vi "Save_Log_File(Subvi).vi"(0 "TX_Station":i32, 1 "RX_Station":i32, 3 "1D data":i32[](array[numeric]) caption="1D 데이터") -> (8 "참조 번호 출력":refnum<file>)   [LabVIEW 2024]
uses:
  <vilib>/Utility/sysdir.llb/System Directory Type.ctl
  <vilib>/Utility/file.llb/Write Delimited Spreadsheet (I64).vi
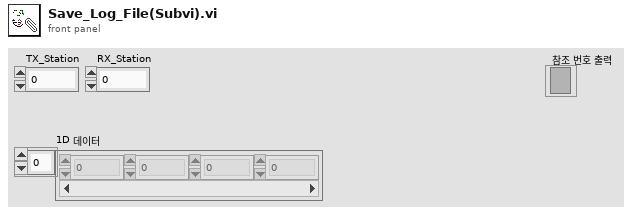
[diagram p1: front panel]
types:
  T1 = enum16{"open", "replace", "create", "open or create", "replace or create", "replace or create with confirmation"}
  T2 = typedef "System Directory Type.ctl" = i32
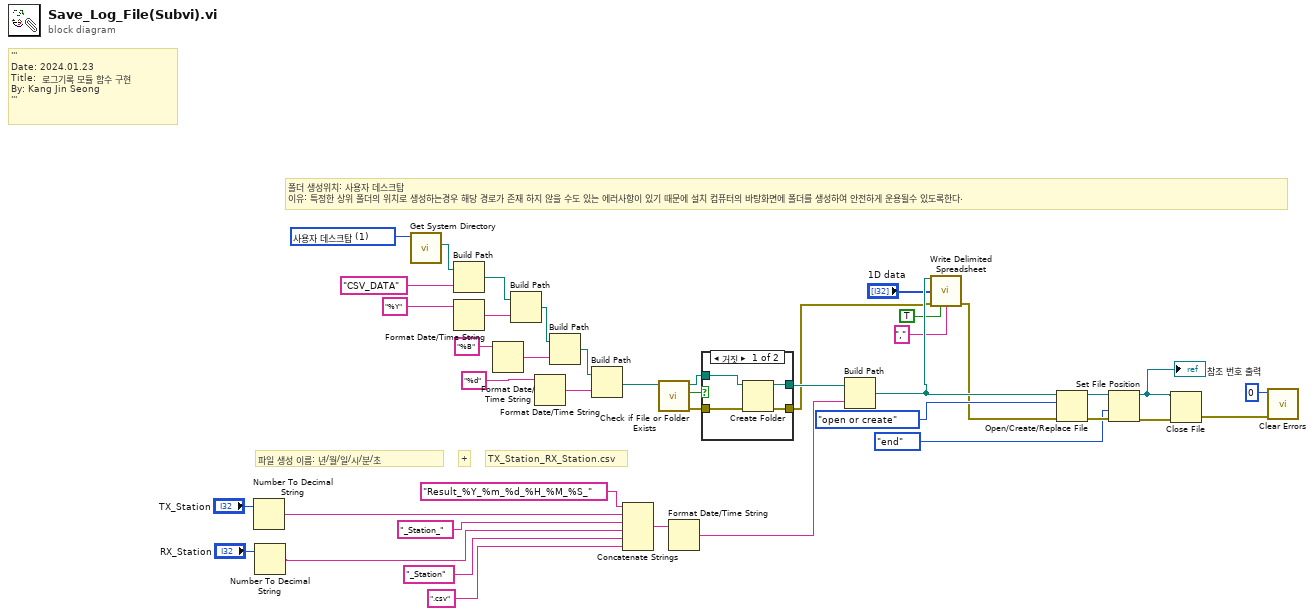
[diagram p0: block diagram]
diagram:
  w35 = T2 1 items=["사용자 홈"=0, "사용자 데스크탑"=1, "사용자 문서"=2, "사용자 어플리케이션 데이터"=3, "사용자 환경"=4, "사용자 임시"=5, "퍼블릭 문서"=6, "퍼블릭 어플리케이션 데이터"=7, "퍼블릭 환경"=8, "퍼블릭 캐시"=13, "시스템 코어 라이브러리"=9, "시스템 설치된 라이브러리"=10, "어플리케이션 파일"=11, "부팅 볼륨 루트"=12] ("system directory type")
  # "+"
  # "TX_Station_RX_Station.csv"
  # "파일 생성 이름: 년/월/일/시/분/초"
  # "폴더 생성위치: 사용자 데스크탑\n이유: 특정한 상위 폴더의 위치로 생성하는경우 해당 경로가 존재 하지 않을 수도 있는 에러사항이 있기 때문에 설치 컴퓨터의 바탕화면에 폴더를 생성하여 안전하게 운용될수 있도록한다."
  # "'''\nDate: 2024.01.23\nTitle:  로그기록 모듈 함수 구현\nBy: Kang Jin Seong\n'''"
  n1 = Number To Decimal String(number="TX_Station") -> (decimal integer string=w10:string)  [unwired: 1 in]
  n2 = Number To Decimal String(number="RX_Station") -> (decimal integer string=w7:string)  [unwired: 1 in]
  n3 = call <vilib>:"Get System Directory.vi"("system directory type"=w35) -> ("system directory"=w41:path)  [unwired: 10 in]
  n4 = Build Path(base path=w41, name or relative path="CSV_DATA") -> (appended path=w29:path)
  n5 = Format Date/Time String(time format string (%c)="%Y") -> (date/time string=w27:string)  [unwired: 2 in]
  n6 = Format Date/Time String(time format string (%c)="%B") -> (date/time string=w26:string)  [unwired: 2 in]
  n7 = Build Path(base path=w29, name or relative path=w27) -> (appended path=w25:path)
  n8 = Format Date/Time String(time format string (%c)="%d") -> (date/time string=w23:string)  [unwired: 2 in]
  n9 = Build Path(base path=w25, name or relative path=w26) -> (appended path=w22:path)
  n10 = Build Path(base path=w22, name or relative path=w23) -> (appended path=w20:path)
  n11 = Concatenate Strings("Result_%Y_%m_%d_%H_%M_%S_" ("시간 포맷 문자열 (%c)"), w10, "_Station_" ("시간 포맷 문자열 (%c)"), w7, "_Station" ("시간 포맷 문자열 (%c)"), ".csv" ("시간 포맷 문자열 (%c)")) -> (w15:string)
  n12 = call <vilib>:"Check if File or Folder Exists.vi"("path"=w20) -> ("error out"=w38:errorcluster, "file or folder exists?"=w40:bool, "dup path"=w39:path)  [unwired: 8 in]
  n13 = Format Date/Time String(time format string (%c)=w15) -> (date/time string=w30:string)  [unwired: 2 in]
  n14 = case shown="거짓" w40 {
    tunnel: w39 -> [w45 w47]
    tunnel: w38 -> [w44 w46]
    tunnel: [w43 w47] -> w31
    tunnel: [w42 w46] -> w4
    frame False {
      n15 = Create Folder(path (use dialog)=w45, error in=w44) -> (created path=w43:path, error out=w42:errorcluster)  [unwired: 1 in, 1 out]
    }
    frame True {
    }
  }
  n16 = Build Path(base path=w31, name or relative path=w30) -> (appended path=w14:path)
  n17 = call-poly <vilib>:"Write Delimited Spreadsheet.vi"("file path (dialog if empty)"=w14, "1D data"="1D data", "error in (no error)"=w4, "transpose? (no:F)"=TRUE, "delimiter (\\t)"="," ("delimiter (\\t)")) -> ("error out"=w3:errorcluster)  [unwired: 9 in, 1 out]
  n18 = Open/Create/Replace File(file path (use dialog)=w14, error in=w3, operation (0:open)=T1."open or create" ("동작(0:open)")) -> (refnum out=w34:refnum<file>, error out=w33:errorcluster)  [unwired: 3 in, 1 out]
  n19 = Set File Position(refnum=w34, from (0:start)=enum16{"start", "end", "current"}."end" ("위치(0:start)"), error in=w33) -> (refnum out=w5:refnum<file>, error out=w6:errorcluster)  [unwired: 1 in]
  "참조 번호 출력" <- w5
  n20 = Close File(refnum=w5, error in=w6) -> (error out=w2:errorcluster)  [unwired: 1 out]
  n21 = call <vilib>:"Clear Errors.vi"("error in (no error)"=w2, "specific error code to clear (0: all)"=0) -> ()  [unwired: 4 in, 2 out]
